vi "FA Number Array.vi"() -> (2 "FA Number String Array":string[](array[string]), 3 "FA Number Array":i32[](array[numeric]))   [LabVIEW 2016, in "M1M3SupportEUI_Views.lvlib"]
uses:
  M1M3SupportEUI_Views.lvlib
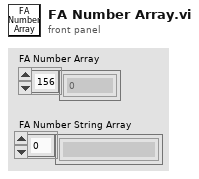
[diagram p1: front panel]
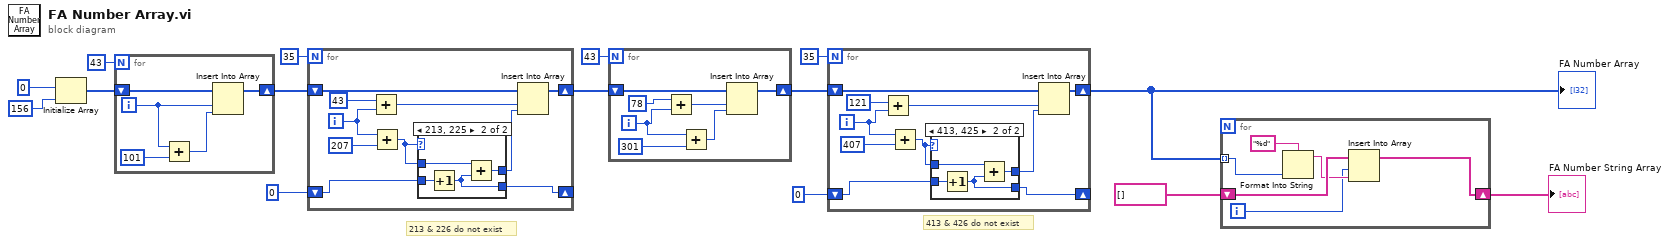
[diagram p0: block diagram]
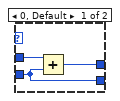
[diagram p2: hidden frame]
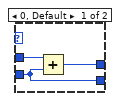
[diagram p3: hidden frame]
diagram:
  # "413 & 426 do not exist"
  # "213 & 226 do not exist"
  n1 = Initialize Array(0, 156 ("dimension size")) -> (w12:i32[])
  n2 = for {
    N: 43 -> [_]
    shift-right: [w18] -> w8
    shift-left: w12 -> [w19]
    i -> [w16]
    n3 = Add(x=w16, y=101) -> (x+y=w20:i32)
    n4 = Insert Into Array(array=w19, index=w16, new element=w20) -> (w18:i32[])
  }
  n5 = for {
    N: 35 -> [_]
    shift-right: [w29] -> w7
    shift-left: w8 -> [w30]
    shift-right: [w21] -> _
    shift-left: 0 -> [w24]
    i -> [w25]
    n6 = Add(x=43, y=w25) -> (x+y=w27:i32)
    n7 = Add(x=w25, y=207) -> (x+y=w23:i32)
    n8 = case shown="213, 225" w23 {
      tunnel: w24 -> [w31 w37]
      tunnel: w23 -> [w33 w35]
      tunnel: [w32 w36] -> w22
      tunnel: [w31 w34] -> w21
      frame 0, Default {
        n9 = Add(x=w33, y=w31) -> (x+y=w32:i32)
      }
      frame 213, 225 {
        n10 = Increment(x=w37) -> (x+1=w34:i32)
        n11 = Add(x=w35, y=w34) -> (x+y=w36:i32)
      }
    }
    n12 = Insert Into Array(array=w30, index=w27, new element=w22) -> (w29:i32[])
  }
  n13 = for {
    N: 43 -> [_]
    shift-right: [w42] -> w6
    shift-left: w7 -> [w43]
    i -> [w39]
    n14 = Add(x=78, y=w39) -> (x+y=w38:i32)
    n15 = Add(x=w39, y=301) -> (x+y=w44:i32)
    n16 = Insert Into Array(array=w43, index=w38, new element=w44) -> (w42:i32[])
  }
  n17 = for {
    N: 35 -> [_]
    shift-right: [w53] -> w1
    shift-left: w6 -> [w54]
    shift-right: [w45] -> _
    shift-left: 0 -> [w46]
    i -> [w51]
    n18 = Add(x=121, y=w51) -> (x+y=w49:i32)
    n19 = Add(x=w51, y=407) -> (x+y=w48:i32)
    n20 = case shown="413, 425" w48 {
      tunnel: w46 -> [w55 w61]
      tunnel: w48 -> [w57 w59]
      tunnel: [w56 w60] -> w47
      tunnel: [w55 w58] -> w45
      frame 0, Default {
        n21 = Add(x=w57, y=w55) -> (x+y=w56:i32)
      }
      frame 413, 425 {
        n22 = Increment(x=w61) -> (x+1=w58:i32)
        n23 = Add(x=w59, y=w58) -> (x+y=w60:i32)
      }
    }
    n24 = Insert Into Array(array=w54, index=w49, new element=w47) -> (w53:i32[])
  }
  "FA Number Array" <- w1
  n25 = for {
    tunnel: w1 -> [w65] mode=indexing
    shift-right: [w66] -> w2
    shift-left: string[] [] -> [w67]
    i -> [w62]
    n26 = Format Into String(format string="%d", w65) -> (resulting string=w63:string)  [unwired: 2 in, 1 out]
    n27 = Insert Into Array(array=w67, index=w62, new element=w63) -> (w66:string[])
  }
  "FA Number String Array" <- w2
